vi "read_user_info.vi"(0 "Authority":u16(ring) items=["学生", "老师"]) -> ()   [LabVIEW 2015]
uses:
  <vilib>/registry/registry.llb/Registry RtKey.ctl
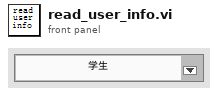
[diagram p1: front panel]
types:
  T1 = typedef "Registry RtKey.ctl" = enum32{"HKEY_CLASSES_ROOT", "HKEY_CURRENT_USER", "HKEY_LOCAL_MACHINE", "HKEY_USERS", "HKEY_PERFORMANCE_DATA", "HKEY_CURRENT_CONFIG", "HKEY_DYN_DATA"}
  T2 = typedef "Registry refnum.ctl" = refnum<k1>
  T3 = cluster{"numSubKeys":i32, "maxSubKeyLen":i32, "maxSubKeyClassLen":i32}
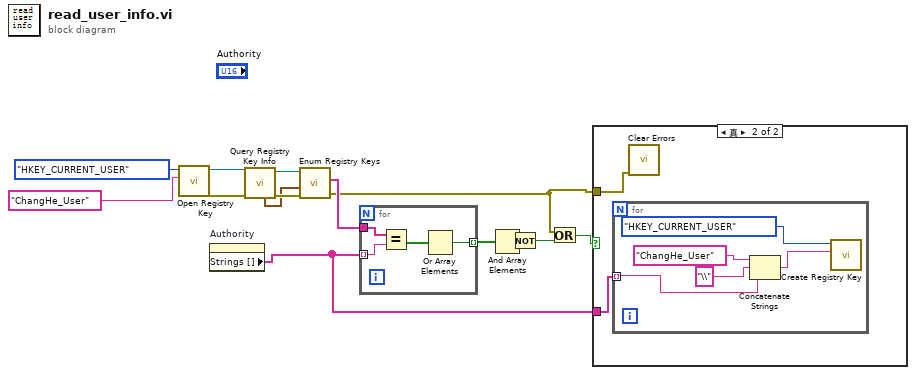
[diagram p0: block diagram]
diagram:
  n1 = call <vilib>:"Open Registry Key.vi"("subkey"="ChangHe_User", "root key (HKEY_LOCAL_MACHINE)"=Registry_RtKey."HKEY_CURRENT_USER") -> ("error out"=w11:errorcluster, "refnum out"=w13:T2)  [unwired: 8 in]
  n2 = property on="Authority" class="Ring (严格)"() -> ("Strings []"=w2:string[])  [unwired: 2 in, 2 out]
  n3 = call <vilib>:"Query Registry Key Info.vi"("error in (no error)"=w11, "refnum"=w13) -> ("error out"=w10:errorcluster, "refnum out"=w9:T2, "subkey info"=w8:T3)  [unwired: 5 in, 2 out]
  n4 = call <vilib>:"Enum Registry Keys.vi"("error in (no error)"=w10, "subkey info"=w8, "refnum"=w9) -> ("error out"=w1:errorcluster, "subkeys"=w7:string[])  [unwired: 6 in, 1 out]
  n5 = for {
    tunnel: w2 -> [w18] mode=indexing
    tunnel: [w16] -> w6 mode=indexing
    tunnel: w7 -> [w15]
    n6 = Equal?(x=w15, y=w18) -> (x = y?=w17:bool[])
    n7 = Or Array Elements(Boolean array=w17) -> (logical OR=w16:bool)
  }
  n8 = And Array Elements(Boolean array=w6) -> (logical AND=w5:bool)
  n9 = Not(x=w5) -> (.not. x?=w4:bool)
  n10 = Or(x=w1, y=w4) -> (x .or. y?=w3:bool)
  n11 = case shown="真" w3 {
    tunnel: w2 -> [_ w19]
    tunnel: w1 -> [_ w20]
    frame False {
    }
    frame True {
      n12 = for {
        tunnel: w19 -> [w22] mode=indexing
        n13 = Concatenate Strings("ChangHe_User" ("subkey"), "\\" ("字符串"), w22) -> (w21:string)
        n14 = call <vilib>:"Create Registry Key.vi"("subkey"=w21, "root key (HKEY_LOCAL_MACHINE)"=Registry_RtKey."HKEY_CURRENT_USER") -> ()  [unwired: 7 in, 3 out]
      }
      n15 = call <vilib>:"Clear Errors.vi"("error in (no error)"=w20) -> ()  [unwired: 5 in, 2 out]
    }
  }
